vi "Configure Dwell Time.vi"(0 "VISA resource name":refnum<visa-resource-name>, 5 "Dwell (1 s)":dbl=1.0 min=0.5 max=999.9 format="%.1f", 11 "error in (no error)":errorcluster) -> (4 "VISA resource name out":refnum<visa-resource-name>, 15 "error out":errorcluster)   [LabVIEW 2016, in "APT 300XAC Series.lvlib"]
doc: "Sets the <B>Dwell time</B> in the power source instrument.\n\n<B>Range</B> : 0.5~999.9 s/m/h\n\nThe dwell parameter configures the actual test time. This time begins after the ramp up and the delay time have completed. The high and low limit thresholds are active during this period."
uses:
  APT 300XAC Series.lvlib
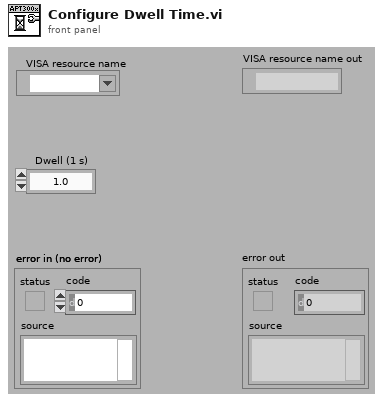
[diagram p1: front panel]
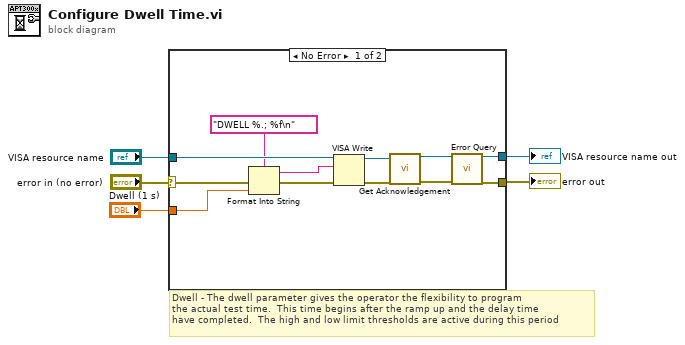
[diagram p0: block diagram]
diagram:
  # "Dwell - The dwell parameter gives the operator the flexibility to program \nthe actual test time.  This time begins after the ramp up and the delay time \nhave completed.  The high and low limit thresholds are active during this period"
  n1 = case shown="No Error" "error in (no error)" {
    selector: "error in (no error)" -> [w11 w19]
    tunnel: "VISA resource name" -> [w17 w18]
    tunnel: [w13 w18] -> w4
    tunnel: [w12 w19] -> w3
    tunnel: "Dwell (1 s)" -> [w16 _]
    frame No Error {
      n2 = Format Into String(format string="DWELL %.; %f\n" ("Command"), error in=w11, w16) -> (resulting string=w15:string, error out=w10:errorcluster)  [unwired: 1 in]
      n3 = VISA Write(VISA resource name=w17, write buffer=w15, error in (no error)=w10) -> (VISA resource name out=w7:refnum<visa-resource-name>, error out=w8:errorcluster)  [unwired: 1 out]
      n4 = call "Get Acknowledgement.vi"("VISA resource name"=w7, "error in (no error)"=w8) -> ("VISA resource name out"=w6:refnum<visa-resource-name>, "error out"=w9:errorcluster)  [unwired: 12 in]
      n5 = call "Error Query.vi"("VISA resource name"=w6, "error in (no error)"=w9) -> ("VISA resource name out"=w13:refnum<visa-resource-name>, "error out"=w12:errorcluster)  [unwired: 10 in, 2 out]
    }
    frame Error {
    }
  }
  "error out" <- w3
  "VISA resource name out" <- w4
